vi "Periodic Tasks.vi"(8 "error in":errorcluster) -> ()   [LabVIEW 2015]
doc: "This VI runs in parallel to other tasks. It can contain as many user-defined periodic loops as you need. These can carry out PID or other sorts of timed response."
uses:
  <vilib>/Rock Robotics/WPI/Utilities/WPI_GetSetVariantRefNum.vi
  Robot Global Data.vi
  <vilib>/Rock Robotics/WPI/Ultrasonic/WPI_SonarMB1010AnalogRefNum Registry Get.vi
  <vilib>/Rock Robotics/WPI/Ultrasonic/WPI_SonarMB1010AnalogGetRange.vi
  <vilib>/Rock Robotics/WPI/RobotDrive/WPI_RobotDriveArcadeDrive_Standard(NoSaturation).vi
panel:
  in  "Intake 2":dbl=-100.0
  in  "Intake":dbl=-100.0
  in  "Shooter RPM":dbl=185.0
  in  "Numeric":dbl=0.2 format="%#_13g"
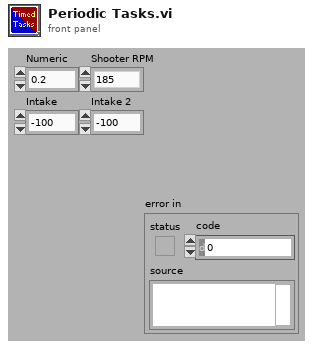
[diagram p1: front panel]
types:
  T1 = typedef "WPI_MotorControlDeviceRef.ctl" = cluster{"DeviceStatus":errorcluster, "Type":T2, "PWM":cluster{"PWM Channel":T3, "DeadBand":T4}, "CAN":cluster{"Device Number":u8, "Control Mode":T5, "Semaphore":T6, "Max Vout":dbl, "TalonSRX Control Mode":T7}, "Invert":bool}
  T2 = typedef "WPI_MotorControlType.ctl" = enum16{"PWM", "CAN", "CANTalonSRX"}
  T3 = typedef "FPGA_DIOPWMChannel.ctl" = enum8{"PWM 0", "PWM 1", "PWM 2", "PWM 3", "PWM 4", "PWM 5", "PWM 6", "PWM 7", "PWM 8", "PWM 9", "PWM MXP 0", "PWM MXP 1", "PWM MXP 2", "PWM MXP 3", "PWM MXP 4", "PWM MXP 5", "PWM MXP 6", "PWM MXP 7", "PWM MXP 8", "PWM MXP 9", "Invalid"}
  T4 = typedef "WPI_PWMDeadband.ctl" = cluster{"Name":string, "maxPositivePwm":i32, "minPositivePwm":i32, "centerPwm":i32, "maxNegativePwm":i32, "minNegativePwm":i32, "angularRange":u16}
  T5 = typedef "WPI_CANJaguar_ControlMode.ctl" = enum8{"Percent VBus", "Current", "Speed", "Position", "Voltage"}
  T6 = typedef "Semaphore RefNum" = refnum<k1>
  T7 = typedef "WPI_CANTalonSRX_APIControlMode.ctl" = enum8{"Percent VBus", "Speed", "Position", "Slave", "Unchanged / Invalid", "Voltage Compensation", "Current", "Motion Profile"}
  T8 = typedef "WPI_JoystickDevRef.ctl" = cluster{"Device":T9}
  T9 = typedef "WPI_JoystickDeviceEnum.ctl" = enum16{"USB 0", "USB 1", "USB 2", "USB 3", "USB 4", "USB 5"}
  T10 = typedef "WPI_SonarMB1010AnalogDeviceRef.ctl" = cluster{"AIDeviceRef":T11, "Scaling factor (V/in)":dbl, "Average Bits":u8}
  T11 = typedef "WPI_AnalogChannelDevRef.ctl" = cluster{"DevStatus":errorcluster, "Analog Channel":T12}
  T12 = typedef "FPGA_AIChannel.ctl" = enum8{"AI 0", "AI 1", "AI 2", "AI 3", "AI MXP 0", "AI MXP 1", "AI MXP 2", "AI MXP 3", "Invalid"}
  T13 = typedef "WPI_GyroDevRef.ctl" = cluster{"DevStatus":errorcluster, "Analog Channel":T12, "Offset":dbl, "Gain (VoltsPerDegree/Second)":dbl, "Gyro Type":enum16{"Analog", "XRS450"}, "Handle":i32, "SPI Bus":T14, "Device Found":bool, "Sample Rate":dbl, "Calibrate On Open":bool}
  T14 = typedef "spi_bus.ctl" = enum16{"SPI On-Board, CS0", "SPI On-Board, CS1", "SPI On-Board, CS2", "SPI On-Board, CS3", "SPI MXP", "Invalid"}
  T15 = typedef "WPI_EncoderDevRef.ctl" = cluster{"DevStatus":errorcluster, "EncoderIndex":T16, "CounterIndex":T17, "DistancePerCount":dbl, "Decoding Type":T18}
  T16 = typedef "FPGA_EncoderIdx.ctl" = enum8{"Enc 0", "Enc 1", "Enc 2", "Enc 3", "Enc 4", "Enc 5", "Enc 6", "Enc 7", "Invalid"}
  T17 = typedef "FPGA_CounterCtrSystemIndex.ctl" = enum8{"Ctr 0", "Ctr 1", "Ctr 2", "Ctr 3", "Ctr 4", "Ctr 5", "Ctr 6", "Ctr 7", "Invalid"}
  T18 = typedef "WPI_EncoderType.ctl" = enum16{"1x", "2x", "4x"}
  T19 = typedef "WPI_RobotDriveDevRef.ctl" = cluster{"DevStatus":errorcluster, "Motors[]":T1[], "Square Inputs":bool, "Max Output":dbl}
  T20 = typedef "WPI_CANTalonSRX_GlobalStatus.ctl" = cluster{"Applied Throttle":dbl, "Module Enabled":bool, "CAN Error":errorcluster, "Closed Loop Error":dbl, "Forward Limit Switch Closed":bool, "Reverse Limit Switch Closed":bool, "Sensor Position":dbl, "Sensor Velocity":dbl, "Current":dbl, "Sticky Fault - Over Temp":bool, "Sticky Fault - Under Voltage":bool, "Sticky Fault - Forward Limit":bool, "Sticky Fault - Reverse Limit":bool, "Sticky Fault - Forward Soft Limit":bool, "Sticky Fault - Reverse Soft Limit":bool, "Brake is Enabled":bool, "Encoder Position":dbl, "Encoder Velocity":dbl, "Encoder Index Count":dbl, "Encoder A Pin State":bool, "Encoder B Pin State":bool, "Encoder Index Pin State":bool, "Analog In":dbl, "Analog In Velocity":dbl, "Temperature (C)":dbl, "Battery Voltage":dbl, "Control 5 Is Supported":bool, "Current Profile Slot Select":dbl, "Pos Div 8":bool, "Vel Div 4":bool, "Pulse Width Position":i32, "Pulse Width Velocity":i32, "Pulse Width Rise To Rise (us)":i32, "Pulse Width Rise To Fall (us)":i32, "Mot Prof Active Is Under Run":bool, "Mot Prof Active Has Under Run":bool, "Mot Prof Active Is Last":bool, "Mot Prof Active Velocity Only":bool, "Mot Prof Active Is Valid":bool, "Mot Prof Buffer Is Full":bool, "Mot Prof Active Profile Slot Select":i32, "Mot Prof NextID":i32, "Mot Prof Count":i32, "Mot Prof Active Velocity":dbl, "Mot Prof Active Position":dbl, "Mot Prof Output Enable":i32}
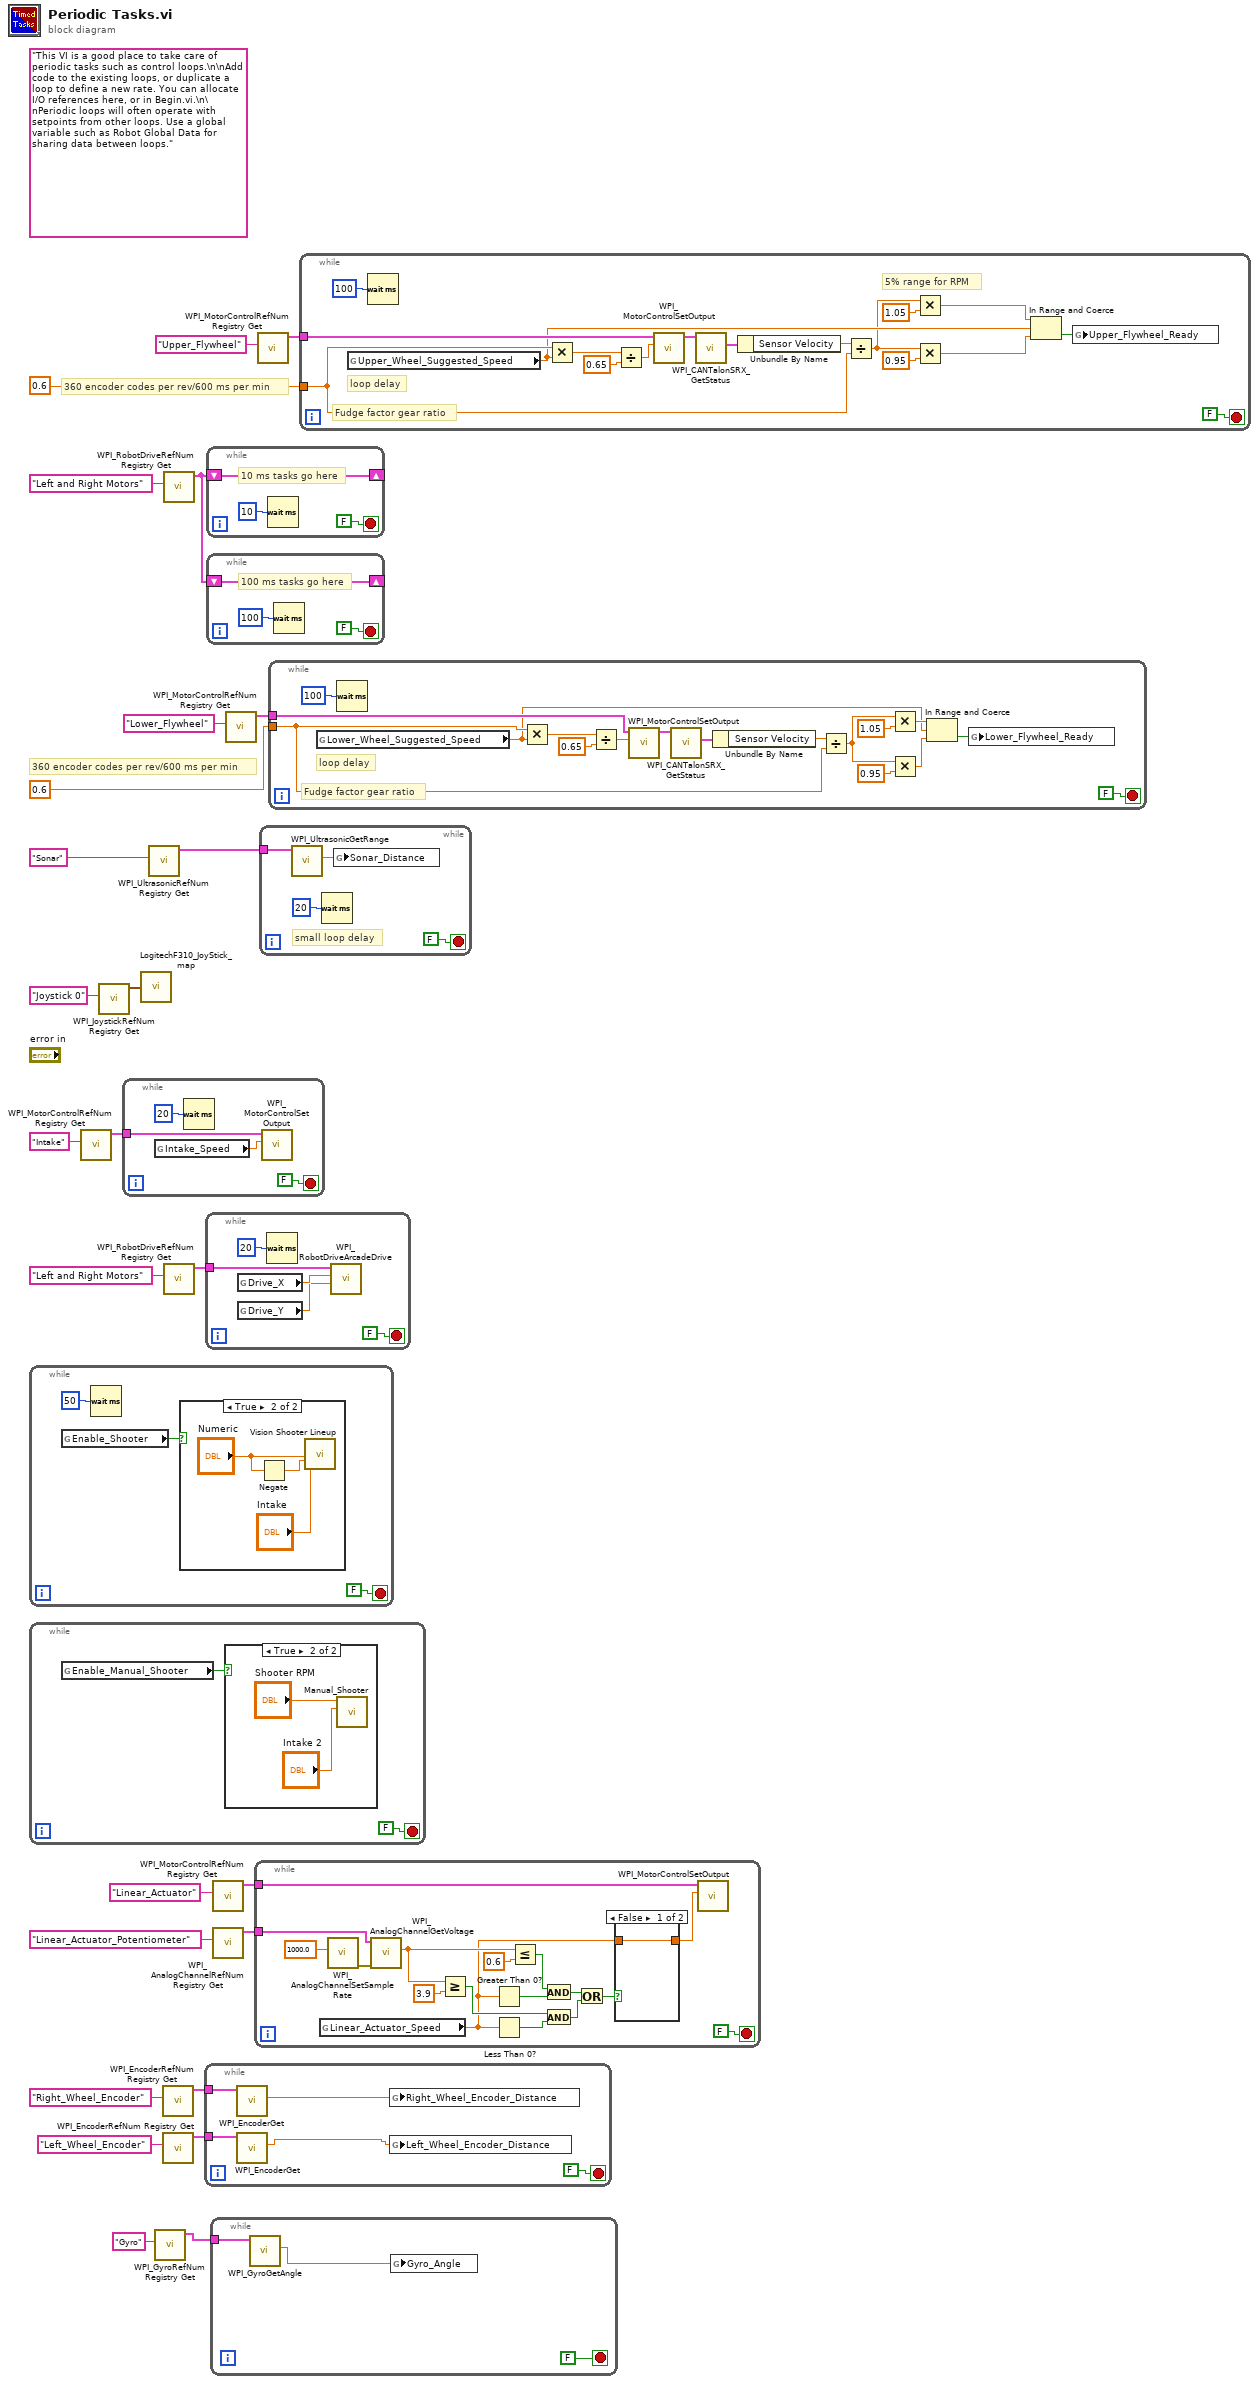
[diagram p0: block diagram]
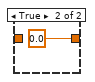
[diagram p2: hidden frame]
diagram:
  (unwired) "This VI is a good place to take care of periodic tasks such as control loops.\n\nAdd code to the existing loops, or duplicate a loop to define a new rate. You can allocate I/O references here, or in Begin.vi.\n\nPeriodic loops will often operate with setpoints from other loops. Use a global variable such as Robot Global Data for sharing data between loops."
  # "360 encoder codes per rev/600 ms per min"
  # "360 encoder codes per rev/600 ms per min"
  n1 = while {
    stop <- FALSE stop-if-true
    n2 = global read "Robot Global Data.vi" "Enable_Shooter"() -> (w29:bool)
    n3 = Wait (ms)(milliseconds to wait=u32 50) -> ()  [unwired: 1 out]
    n4 = case shown="True" w29 {
      frame False {
      }
      frame True {
        n5 = Negate(x="Numeric") -> (-x=w31:dbl)
        n6 = call "Vision Shooter Lineup.vi"("X axis value"="Numeric", "X axis value 2"=w31, "Intake"="Intake") -> ()  [unwired: 25 in]
      }
    }
  }
  n7 = while {
    stop <- FALSE stop-if-true
    n8 = global read "Robot Global Data.vi" "Enable_Manual_Shooter"() -> (w34:bool)
    n9 = case shown="True" w34 {
      frame False {
      }
      frame True {
        n10 = call "Manual_Shooter.vi"("Intake"="Intake 2", "Shooter RPM"="Shooter RPM") -> ()  [unwired: 10 in]
      }
    }
  }
  n11 = call <vilib>:"WPI_MotorControlRefNum Registry Get.vi"("refnum name"="Intake") -> ("MotorControlDevRef"=w13:T1)  [unwired: 9 in, 1 out]
  n12 = call <vilib>:"WPI_JoystickRefNum Registry Get.vi"("refnum name"="Joystick 0") -> ("JoystickDevRef"=w23:T8)  [unwired: 1 in, 9 out]
  n13 = while {
    tunnel: w13 -> [w39]
    stop <- FALSE stop-if-true
    n14 = global read "Robot Global Data.vi" "Intake_Speed"() -> (w38:dbl)
    n15 = Wait (ms)(milliseconds to wait=u32 20) -> ()  [unwired: 1 out]
    n16 = call <vilib>:"WPI_MotorControlSetOutput.vi"("Output"=w38, "MotorControlDevRef"=w39) -> ()  [unwired: 7 in, 3 out]
  }
  n17 = call "LogitechF310_JoyStick_map.vi"("JoystickDevRef"=w23) -> ()  [unwired: 2 out]
  n18 = call-poly <vilib>:"WPI_UltrasonicRefNum Registry Get.vi"("refnum name"="Sonar") -> ("SonarMB1010AnalogDevRef"=w16:T10)  [unwired: 9 in, 1 out]
  n19 = call <vilib>:"WPI_GyroRefNum Registry Get.vi"("refnum name"="Gyro") -> ("GyroDevRef"=w1:T13)  [unwired: 9 in, 1 out]
  n20 = call <vilib>:"WPI_EncoderRefNum Registry Get.vi"("refnum name"="Right_Wheel_Encoder") -> ("EncoderDevRef"=w3:T15)  [unwired: 9 in, 1 out]
  n21 = call <vilib>:"WPI_EncoderRefNum Registry Get.vi"("refnum name"="Left_Wheel_Encoder") -> ("EncoderDevRef"=w4:T15)  [unwired: 9 in, 1 out]
  n22 = call <vilib>:"WPI_RobotDriveRefNum Registry Get.vi"("refnum name"="Left and Right Motors") -> ("RobotDriveDevRef"=w24:T19)  [unwired: 1 in, 9 out]
  n23 = call <vilib>:"WPI_RobotDriveRefNum Registry Get.vi"("refnum name"="Left and Right Motors") -> ("RobotDriveDevRef"=w11:T19)  [unwired: 9 in, 1 out]
  n24 = while {
    tunnel: w4 -> [w45]
    tunnel: w3 -> [w44]
    stop <- FALSE stop-if-true
    n25 = call <vilib>:"WPI_EncoderGet.vi"("EncoderDevRef"=w44) -> ("Distance"=w41:dbl)  [unwired: 5 in, 5 out]
    n26 = call <vilib>:"WPI_EncoderGet.vi"("EncoderDevRef"=w45) -> ("Distance"=w42:dbl)  [unwired: 5 in, 5 out]
    n27 = global write "Robot Global Data.vi" "Right_Wheel_Encoder_Distance"(w41) -> ()
    n28 = global write "Robot Global Data.vi" "Left_Wheel_Encoder_Distance"(w42) -> ()
  }
  n29 = while {
    tunnel: w11 -> [w48]
    stop <- FALSE stop-if-true
    n30 = global read "Robot Global Data.vi" "Drive_X"() -> (w50:dbl)
    n31 = global read "Robot Global Data.vi" "Drive_Y"() -> (w49:dbl)
    n32 = Wait (ms)(milliseconds to wait=u32 20) -> ()  [unwired: 1 out]
    n33 = call-poly <vilib>:"WPI_RobotDriveArcadeDrive.vi"("Y axis value"=w49, "X axis value"=w50, "RobotDriveDevRef"=w48) -> ()  [unwired: 6 in, 3 out]
  }
  n34 = while {
    shift-right: [w51] -> _
    shift-left: w24 -> [w51]
    stop <- FALSE stop-if-true
    # "10 ms tasks go here"
    n35 = Wait (ms)(milliseconds to wait=u32 10) -> ()  [unwired: 1 out]
  }
  n36 = while {
    shift-right: [w54] -> _
    shift-left: w24 -> [w54]
    stop <- FALSE stop-if-true
    # "100 ms tasks go here"
    n37 = Wait (ms)(milliseconds to wait=u32 100) -> ()  [unwired: 1 out]
  }
  n38 = while {
    tunnel: w1 -> [w59]
    stop <- FALSE stop-if-true
    n39 = call <vilib>:"WPI_GyroGetAngle.vi"("GyroDevRef"=w59) -> ("Angle"=w58:dbl)  [unwired: 6 in, 4 out]
    n40 = global write "Robot Global Data.vi" "Gyro_Angle"(w58) -> ()
  }
  n41 = call <vilib>:"WPI_MotorControlRefNum Registry Get.vi"("refnum name"="Linear_Actuator") -> ("MotorControlDevRef"=w7:T1)  [unwired: 9 in, 1 out]
  n42 = call <vilib>:"WPI_AnalogChannelRefNum Registry Get.vi"("refnum name"="Linear_Actuator_Potentiometer") -> ("AIDeviceRef"=w9:T11)  [unwired: 9 in, 1 out]
  n43 = call <vilib>:"WPI_MotorControlRefNum Registry Get.vi"("refnum name"="Lower_Flywheel") -> ("MotorControlDevRef"=w19:T1)  [unwired: 9 in, 1 out]
  n44 = while {
    tunnel: w9 -> [w76]
    tunnel: w7 -> [w75]
    stop <- FALSE stop-if-true
    n45 = global read "Robot Global Data.vi" "Linear_Actuator_Speed"() -> (w63:dbl)
    n46 = call <vilib>:"WPI_AnalogChannelSetSampleRate.vi"("Samples Per Second (per channel)"=1000.0) -> ("error out"=w62:errorcluster)  [unwired: 4 in, 6 out]
    n47 = call <vilib>:"WPI_AnalogChannelGetVoltage.vi"("error in (no error)"=w62, "AIDeviceRef"=w76) -> ("Voltage"=w65:dbl)  [unwired: 7 in, 2 out]
    n48 = Greater Or Equal?(x=w65, y=3.9) -> (x >= y?=w72:bool)
    n49 = Greater Than 0?(x=w63) -> (x > 0?=w67:bool)
    n50 = Less Than 0?(x=w63) -> (x < 0?=w73:bool)
    n51 = Less Or Equal?(x=w65, y=0.6) -> (x <= y?=w68:bool)
    n52 = And(x=w68, y=w67) -> (x .and. y?=w66:bool)
    n53 = And(x=w72, y=w73) -> (x .and. y?=w71:bool)
    n54 = Or(x=w66, y=w71) -> (x .or. y?=w70:bool)
    n55 = case shown="False" w70 {
      tunnel: w63 -> [w77 _]
      tunnel: [w77 0.0] -> w64
      frame False {
      }
      frame True {
      }
    }
    n56 = call <vilib>:"WPI_MotorControlSetOutput.vi"("Output"=w64, "MotorControlDevRef"=w75) -> ()  [unwired: 7 in, 3 out]
  }
  n57 = call <vilib>:"WPI_MotorControlRefNum Registry Get.vi"("refnum name"="Upper_Flywheel") -> ("MotorControlDevRef"=w22:T1)  [unwired: 9 in, 1 out]
  n58 = while {
    tunnel: w16 -> [w81]
    stop <- FALSE stop-if-true
    # "small loop delay"
    n59 = call-poly <vilib>:"WPI_UltrasonicGetRange.vi"("SonarMB1010AnalogDevRef"=w81) -> ("Distance"=w79:dbl)  [unwired: 8 in, 2 out]
    n60 = Wait (ms)(milliseconds to wait=u32 20) -> ()  [unwired: 1 out]
    n61 = global write "Robot Global Data.vi" "Sonar_Distance"(w79) -> ()
  }
  n62 = while {
    tunnel: w19 -> [w91]
    tunnel: 0.6 ("x") -> [w90]
    stop <- FALSE ("stop") stop-if-true
    # "Fudge factor gear ratio"
    # "loop delay"
    n63 = global read "Robot Global Data.vi" "Lower_Wheel_Suggested_Speed"() -> (w85:dbl)
    n64 = Wait (ms)(milliseconds to wait=u32 100) -> ()  [unwired: 1 out]
    n65 = Multiply(x=w90, y=w85) -> (x*y=w95:dbl)
    n66 = Divide(x=w95, y=0.65 ("x")) -> (x/y=w93:dbl)
    n67 = call <vilib>:"WPI_MotorControlSetOutput.vi"("Output"=w93, "MotorControlDevRef"=w91) -> ("MotorControlDevRef"=w98:T1)  [unwired: 7 in, 2 out]
    n68 = call <vilib>:"WPI_CANTalonSRX_GetStatus.vi"("CAN Talon SRX Ref"=w98) -> ("Talon SRX Status"=w97:T20)  [unwired: 8 in, 2 out]
    n69 = Unbundle By Name(w97) -> ("Sensor Velocity"=w96:dbl)
    n70 = Divide(x=w96, y=w90) -> (x/y=w84:dbl)
    n71 = Multiply(x=w84, y=1.05) -> (x*y=w88:dbl)
    n72 = Multiply(x=w84, y=0.95) -> (x*y=w86:dbl)
    n73 = In Range and Coerce(upper limit=w88, x=w85, lower limit=w86) -> (In Range?=w83:bool)  [unwired: 1 out]
    n74 = global write "Robot Global Data.vi" "Lower_Flywheel_Ready"(w83) -> ()
  }
  n75 = while {
    tunnel: w22 -> [w108]
    tunnel: 0.6 ("x") -> [w107]
    stop <- FALSE ("stop") stop-if-true
    # "5% range for RPM"
    # "Fudge factor gear ratio"
    # "loop delay"
    n76 = global read "Robot Global Data.vi" "Upper_Wheel_Suggested_Speed"() -> (w102:dbl)
    n77 = Wait (ms)(milliseconds to wait=u32 100) -> ()  [unwired: 1 out]
    n78 = Multiply(x=w107, y=w102) -> (x*y=w112:dbl)
    n79 = Divide(x=w112, y=0.65 ("x")) -> (x/y=w110:dbl)
    n80 = call <vilib>:"WPI_MotorControlSetOutput.vi"("Output"=w110, "MotorControlDevRef"=w108) -> ("MotorControlDevRef"=w115:T1)  [unwired: 7 in, 2 out]
    n81 = call <vilib>:"WPI_CANTalonSRX_GetStatus.vi"("CAN Talon SRX Ref"=w115) -> ("Talon SRX Status"=w114:T20)  [unwired: 8 in, 2 out]
    n82 = Unbundle By Name(w114) -> ("Sensor Velocity"=w113:dbl)
    n83 = Divide(x=w113, y=w107) -> (x/y=w101:dbl)
    n84 = Multiply(x=w101, y=1.05) -> (x*y=w105:dbl)
    n85 = Multiply(x=w101, y=0.95) -> (x*y=w103:dbl)
    n86 = In Range and Coerce(upper limit=w105, x=w102, lower limit=w103) -> (In Range?=w100:bool)  [unwired: 1 out]
    n87 = global write "Robot Global Data.vi" "Upper_Flywheel_Ready"(w100) -> ()
  }
